vi "Populate Attr XML Priv.vi"(0 "Attribute Names":string[](array[string]), 2 "Data Types Dict":variant, 5 "Attribute Values":variant[](array[variant]), 13 "Indent":i32) -> (4 "Attr XML Strings":string[](array[string]))   [LabVIEW 2017, in "Tree API.lvlib" / "Tree.lvclass"]
uses:
  Tree.lvclass
  Tree Data/Tree Data.lvclass
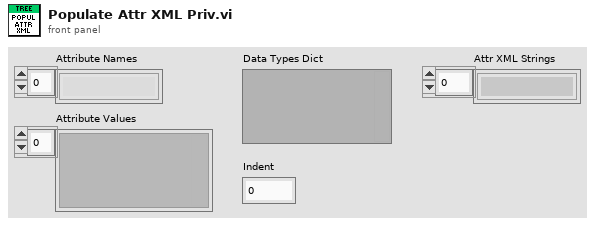
[diagram p1: front panel]
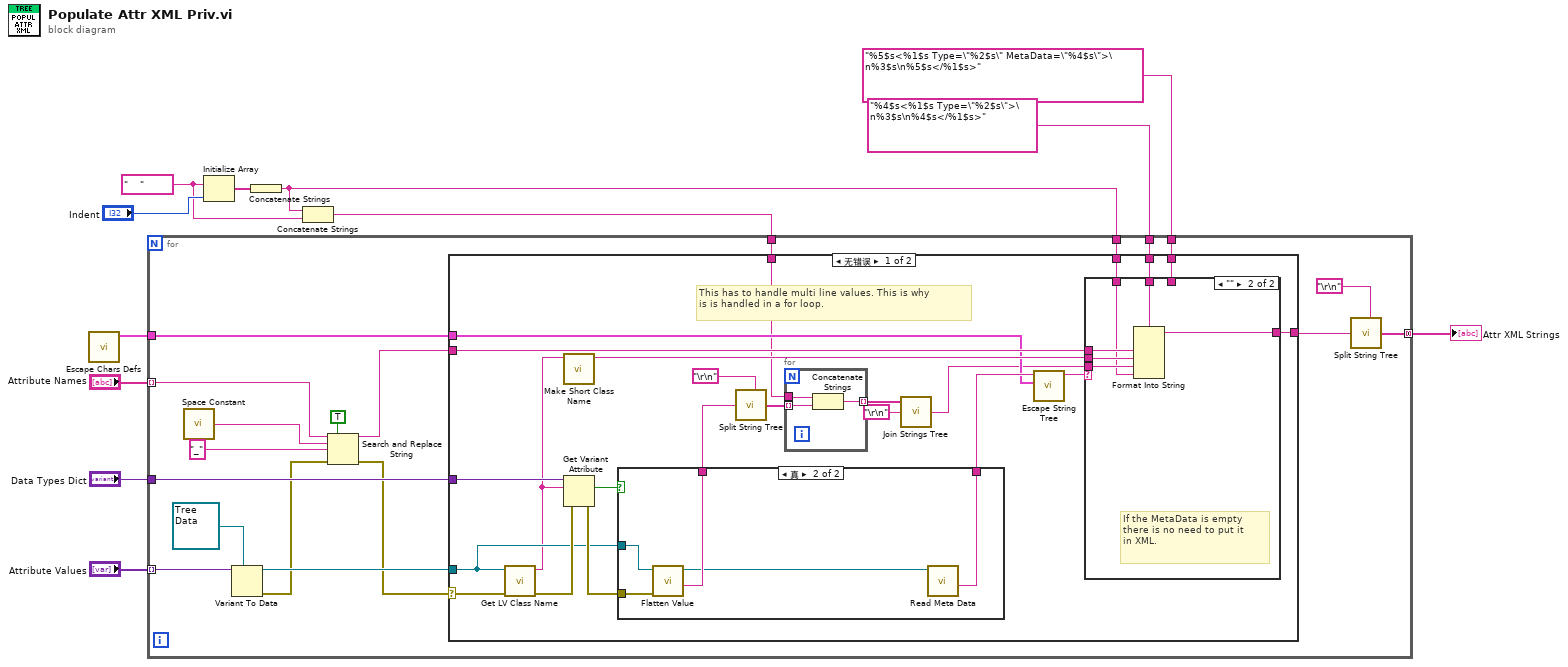
[diagram p0: block diagram]
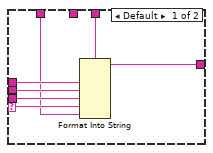
[diagram p3: hidden frame]
diagram:
  w3 = "    "
  n1 = call "Escape Chars Defs.vi"() -> ("Escapes"=w7:cluster{"String":string, "Escape":string}[])  [unwired: 11 in]
  n2 = Initialize Array(w3, "Indent") -> (w6:string[])
  n3 = Concatenate Strings(w6) -> (w1:string)
  n4 = Concatenate Strings(w1, w3) -> (w2:string)
  n5 = for {
    tunnel: "Attribute Names" -> [w19] mode=indexing
    tunnel: "Attribute Values" -> [w31] mode=indexing
    tunnel: "Data Types Dict" -> [w29]
    tunnel: "%5$s<%1$s Type=\"%2$s\" MetaData=\"%4$s\">\n%3$s\n%5$s</%1$s>" ("format string") -> [w27]
    tunnel: "%4$s<%1$s Type=\"%2$s\">\n%3$s\n%4$s</%1$s>" ("format string") -> [w26]
    tunnel: [w15] -> w4 mode=concatenating
    tunnel: w7 -> [w25]
    tunnel: w2 -> [w14]
    tunnel: w1 -> [w13]
    n6 = call <vilib>:"Space Constant.vi"() -> ("String"=w24:string)
    n7 = Variant To Data(type=refnum<class "Tree Data.lvclass"> refnum ("Tree Data.lvclass"), Variant=w31) -> (data=w30:refnum<class "Tree Data.lvclass">, error out=w21:errorcluster)  [unwired: 1 in]
    n8 = Search and Replace String(replace all?=TRUE ("replace all? (F)"), input string=w19, search string=w24, replace string="_", error in=w21) -> (result string=w18:string, error out=w20:errorcluster)  [unwired: 3 in, 2 out]
    n9 = case shown="无错误" w20 {
      selector: w20 -> [w54 _]
      tunnel: w30 -> [w49 _]
      tunnel: w18 -> [w48 _]
      tunnel: w29 -> [w53 _]
      tunnel: w27 -> [w47 _]
      tunnel: w26 -> [w46 _]
      tunnel: [w44 _] -> w17
      tunnel: w25 -> [w40 _]
      tunnel: w14 -> [w36 _]
      tunnel: w13 -> [w32 _]
      frame No Error {
        # "This has to handle multi line values. This is why\nis is handled in a for loop."
        n10 = call <vilib>:"Get LV Class Name.vi"("error in (no error)"=w54, "object"=w49) -> ("error out"=w52:errorcluster, "class name"=w45:string)  [unwired: 8 in]
        n11 = call "Make Short Class Name.vi"("Class Name"=w45) -> ("Shortened Class Name"=w43:string)  [unwired: 10 in]
        n12 = Get Variant Attribute(Variant=w53, name=w45, error in=w52) -> (found=w50:bool, error out=w51:errorcluster)  [unwired: 1 in, 2 out]
        n13 = case shown="真" w50 {
          tunnel: [_ w62] -> w39
          tunnel: [_ w58] -> w42
          tunnel: w51 -> [_ w59]
          tunnel: w49 -> [_ w60]
          frame False {
          }
          frame True {
            n14 = call-dynamic "Flatten Value.vi"("Error In"=w59, "Tree Data In"=w60) -> ("Value"=w62:string, "Tree Data Out"=w61:refnum<class "Tree Data.lvclass">)  [unwired: 7 in, 1 out]
            n15 = call "Read Meta Data.vi"("Tree Data In"=w61) -> ("Meta Data"=w58:string)  [unwired: 9 in, 1 out]
          }
        }
        n16 = call "Split String Tree.vi"("Split Pattern"="\r\n", "Input String"=w39) -> ("Split String"=w37:string[])  [unwired: 5 in]
        n17 = for {
          tunnel: w37 -> [w57] mode=indexing
          tunnel: w36 -> [w56]
          tunnel: [w55] -> w35 mode=indexing
          n18 = Concatenate Strings(w56, w57) -> (w55:string)
        }
        n19 = call "Join Strings Tree.vi"("Separator (,)"="\r\n", "Strings In"=w35) -> ("String"=w33:string)  [unwired: 1 in]
        n20 = call "Escape String Tree.vi"("Escapes"=w40, "String In"=w42) -> ("String Out"=w41:string)  [unwired: 9 in]
        n21 = case shown="\"\"" w41 {
          selector: w41 -> [w65 _]
          tunnel: w43 -> [w67 w73]
          tunnel: w48 -> [w66 w74]
          tunnel: w47 -> [w69 _]
          tunnel: w33 -> [w68 w72]
          tunnel: w46 -> [_ w75]
          tunnel: [w64 w71] -> w44
          tunnel: w32 -> [w63 w70]
          frame Default {
            n22 = Format Into String(format string=w69, w66, w67, w68, w65, w63) -> (resulting string=w64:string)  [unwired: 2 in, 1 out]
          }
          frame "" {
            # "If the MetaData is empty\nthere is no need to put it\nin XML."
            n23 = Format Into String(format string=w75, w74, w73, w72, w70) -> (resulting string=w71:string)  [unwired: 2 in, 1 out]
          }
        }
      }
      frame Error {
      }
    }
    n24 = call "Split String Tree.vi"("Split Pattern"="\r\n", "Input String"=w17) -> ("Split String"=w15:string[])  [unwired: 5 in]
  }
  "Attr XML Strings" <- w4
